vi "pointBehindBallToStealBall.vi"(8 "distanceBehindBallToStealBall":dbl=400.0, 9 "Field":refnum<class "Field.lvclass">, 10 "Ball":refnum<class "Ball.lvclass">, 11 "Robot in":refnum<class "Robot.lvclass">) -> (2 "pointBehindBall":dbl[](array[numeric]))   [LabVIEW 2021, in "StealBallSkill.lvclass"]
uses:
  StealBallSkill.lvclass
  Robot_class/Robot.lvclass
  Field_class/Field.lvclass
  Ball_class/Ball.lvclass
  D:/RoboIme/horie/SSL_AI/Object_class/Object.lvclass
  Object_class/Object.lvclass/Object.ctl
  <vilib>/Analysis/baseanly.llb/Unit Vector (DBL).vi
  Object_class/Read position(x,y).vi
  <vilib>/Analysis/NI_AALBase.lvlib
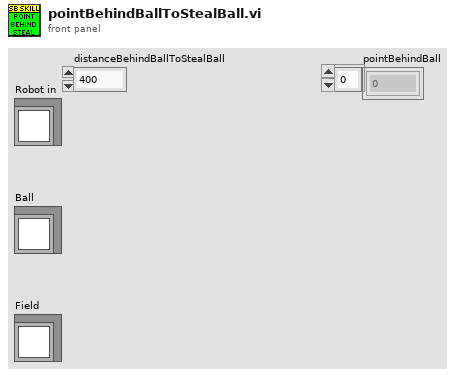
[diagram p1: front panel]
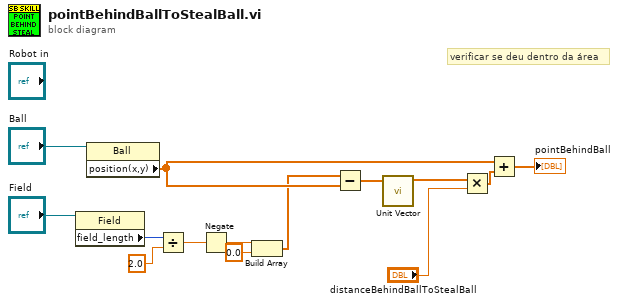
[diagram p0: block diagram]
diagram:
  # "verificar se deu dentro da área"
  n1 = property class="Field"(reference="Field") -> ("field_length"=w5:i32)  [unwired: 1 in, 2 out]
  n2 = property class="Ball"(reference="Ball") -> ("position(x,y)"=w12:dbl[])  [unwired: 1 in, 2 out]
  n3 = Divide(x=w5, y=2.0) -> (x/y=w7:dbl)
  n4 = Negate(x=w7) -> (-x=w8:dbl)
  n5 = Build Array(w8, 0.0 ("element")) -> (w10:dbl[])
  n6 = Subtract(x=w10, y=w12) -> (x-y=w11:dbl[])
  n7 = call-poly <vilib>:"Unit Vector.vi"("Input Vector"=w11) -> ("Unit Vector"=w14:dbl[])  [unwired: 8 in, 2 out]
  n8 = Multiply(x=w14, y="distanceBehindBallToStealBall") -> (x*y=w13:dbl[])
  n9 = Add(x=w12, y=w13) -> (x+y=→"pointBehindBall":dbl[])
